vi "Get_Drive_Commands.vi"(9 "Rotation Multiplier":dbl, 10 "Strafe Multiplier":dbl, 11 "Driver Inputs":T2) -> (3 "Drive Command Inputs":T1)   [LabVIEW 2012]
uses:
  Joystick_Inputs.ctl
  <vilib>/Rock Robotics/WPI/Joystick/WPI_JoystickButtonState.ctl
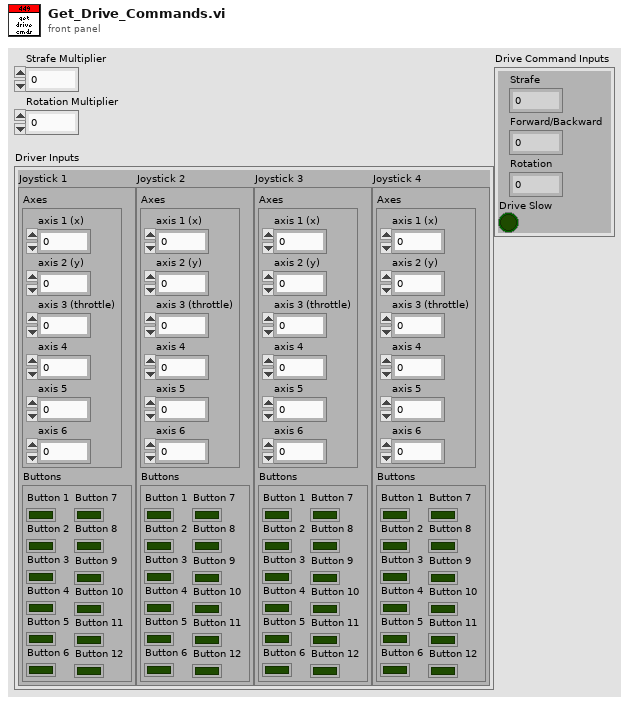
[diagram p1: front panel]
types:
  T1 = cluster{"Strafe":dbl, "Forward/Backward":dbl, "Rotation":dbl, "Drive Slow":bool}
  T2 = typedef "Joystick_Inputs.ctl" = cluster{"Joystick 1":cluster{"Axes":cluster{"axis 1 (x)":dbl, "axis 2 (y)":dbl, "axis 3 (throttle)":dbl, "axis 4":dbl, "axis 5":dbl, "axis 6":dbl}, "Buttons":T3}, "Joystick 2":cluster{"Axes":cluster{"axis 1 (x)":dbl, "axis 2 (y)":dbl, "axis 3 (throttle)":dbl, "axis 4":dbl, "axis 5":dbl, "axis 6":dbl}, "Buttons":T3}, "Joystick 3":cluster{"Axes":cluster{"axis 1 (x)":dbl, "axis 2 (y)":dbl, "axis 3 (throttle)":dbl, "axis 4":dbl, "axis 5":dbl, "axis 6":dbl}, "Buttons":T3}, "Joystick 4":cluster{"Axes":cluster{"axis 1 (x)":dbl, "axis 2 (y)":dbl, "axis 3 (throttle)":dbl, "axis 4":dbl, "axis 5":dbl, "axis 6":dbl}, "Buttons":T3}}
  T3 = typedef "WPI_JoystickButtonState.ctl" = cluster{"Button 1":bool, "Button 2":bool, "Button 3":bool, "Button 4":bool, "Button 5":bool, "Button 6":bool, "Button 7":bool, "Button 8":bool, "Button 9":bool, "Button 10":bool, "Button 11":bool, "Button 12":bool}
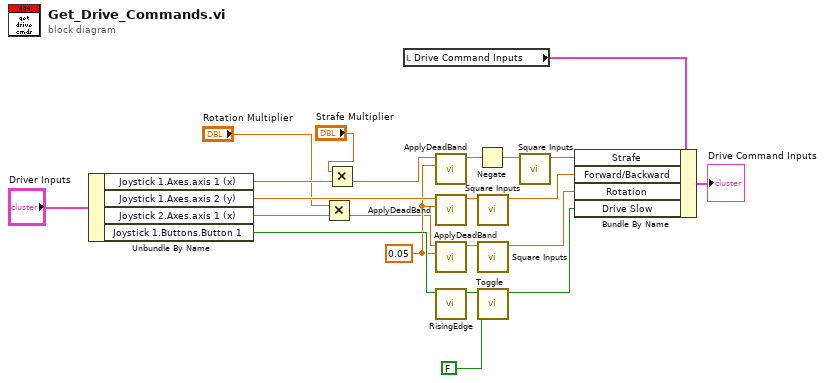
[diagram p0: block diagram]
diagram:
  w6 = 0.05 ("Deadband")
  n1 = Unbundle By Name("Driver Inputs") -> ("Joystick 1.Axes.axis 1 (x)"=w9:dbl, "Joystick 1.Axes.axis 2 (y)"=w8:dbl, "Joystick 2.Axes.axis 1 (x)"=w7:dbl, "Joystick 1.Buttons.Button 1"=w20:bool)
  n2 = Multiply(x="Rotation Multiplier", y=w7) -> (x*y=w5:dbl)
  n3 = Multiply(x="Strafe Multiplier", y=w9) -> (x*y=w4:dbl)
  n4 = local read "Drive Command Inputs"() -> (w21:T1)
  n5 = call "ApplyDeadBand.vi"("Deadband"=w6, "Input"=w4) -> ("Input with deadband"=w12:dbl)  [unwired: 9 in]
  n6 = call "ApplyDeadBand.vi"("Deadband"=w6, "Input"=w8) -> ("Input with deadband"=w11:dbl)  [unwired: 9 in]
  n7 = call "ApplyDeadBand.vi"("Deadband"=w6, "Input"=w5) -> ("Input with deadband"=w10:dbl)  [unwired: 9 in]
  n8 = call "RisingEdge.vi"("BooleanIn"=w20) -> ("BooleanOut"=w13:bool)  [unwired: 10 in]
  n9 = Negate(x=w12) -> (-x=w15:dbl)
  n10 = call "Square Inputs.vi"("Input"=w11) -> ("Squared Value"=w18:dbl)  [unwired: 10 in]
  n11 = call "Square Inputs.vi"("Input"=w10) -> ("Squared Value"=w19:dbl)  [unwired: 10 in]
  n12 = call "Toggle.vi"("Initial"=FALSE, "Toggle"=w13) -> ("BoolOut"=w14:bool)  [unwired: 9 in]
  n13 = call "Square Inputs.vi"("Input"=w15) -> ("Squared Value"=w17:dbl)  [unwired: 10 in]
  n14 = Bundle By Name(cluster=w21, "Strafe"=w17, "Forward/Backward"=w18, "Rotation"=w19, "Drive Slow"=w14) -> (→"Drive Command Inputs":T1)
